vi "niScope Multi Fetch Binary 8.vi"(7 "timeout":dbl=5.0 format="%.2f", 8 "error in":errorcluster, 9 "numSamples":i32=-1, 10 "channels":string="0", 11 "instrument handle":refnum<k15>) -> (0 "error out":errorcluster, 1 "wfm":i8[][](array[numeric]), 2 "wfm info":T1(array[cluster]) {"reserved2" format="%.2f"; "reserved1" format="%.2f"; "offset" format="%^.3e"; "gain" format="%^.3e"; "xIncrement" format="%^.3e"; "relativeInitialX" format="%^.3e"; "absoluteInitialX" format="%^.3e"}, 3 "instrument handle out":refnum<k15>)   [LabVIEW 2020]
doc: "Retrieves data from multiple channels and records. Returns a two-dimensional array of binary 8-bit waveforms."
uses:
  niScope_32.dll
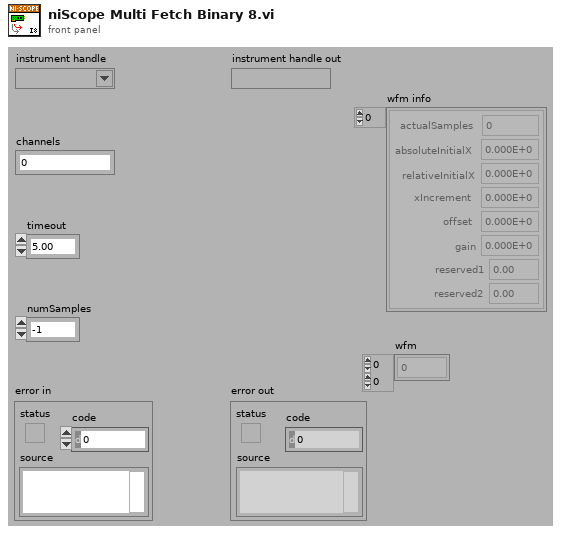
[diagram p1: front panel]
types:
  T1 = cluster{"actualSamples":i32, "absoluteInitialX":dbl, "relativeInitialX":dbl, "xIncrement":dbl, "offset":dbl, "gain":dbl, "reserved1":dbl, "reserved2":dbl}[]
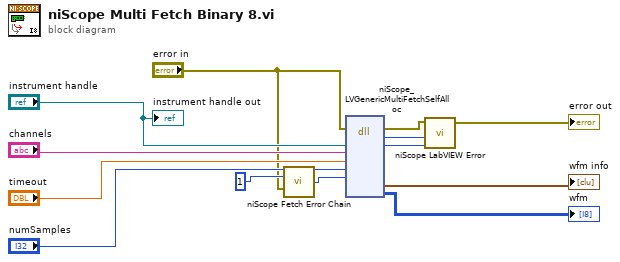
[diagram p0: block diagram]
diagram:
  n1 = call "niScope Fetch Error Chain.vi"("dataType in"=1 ("dataType"), "error in"="error in") -> ("dataType"=w3:i32)  [unwired: 13 in]
  n2 = dll-call lib="niScope_*.*" fn="niScope_LVGenericMultiFetchSelfAlloc"(error in="error in", "instrument handle"="instrument handle", "channelList"="channels", "timeout"="timeout", "numSamples"="numSamples", "dataType"=w3) -> (error out=w1:errorcluster, "status"=w5:i32, "instrument handle"=w4:u32, "wfm info"=→"wfm info":T1, "wfm"=→"wfm":i8[][])  [unwired: 8 in, 1 out]
  n3 = call "niScope LabVIEW Error.vi"("instrument handle"=w4, "niScope error code (0)"=w5, "error in (no error)"=w1) -> ("error out"=→"error out":errorcluster)  [unwired: 2 in]
  "instrument handle out" <- "instrument handle"
